vi "Get Project Paths.vi"(8 "error in (no error)":errorcluster, 11 "VI in":refnum<vi>) -> (0 "error out":errorcluster, 1 "project errors path":path, 2 "project path":path, 3 "VI out":refnum<vi>)   [LabVIEW 2017]
doc: "Returns <b>project path</b> for the <b>VI in</b> owning project and project errors file path if such file exist. Errors file name format is: project_name-errors.txt"
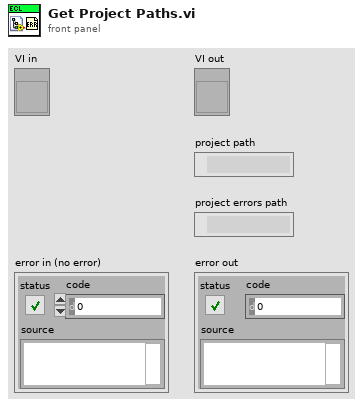
[diagram p1: front panel]
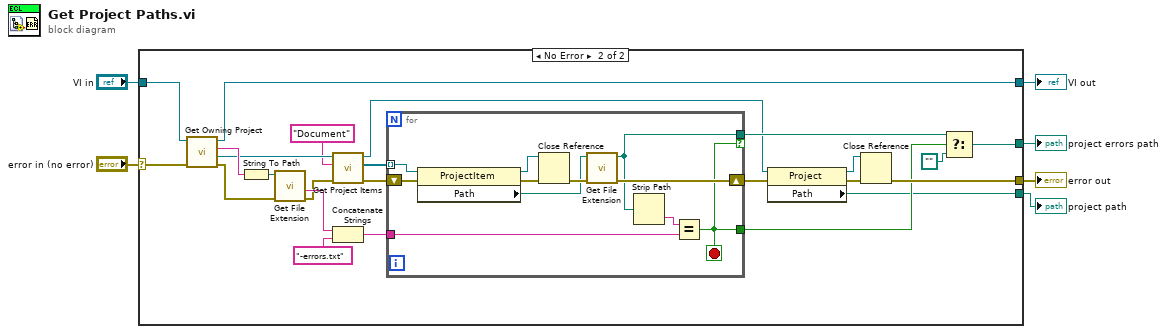
[diagram p0: block diagram]
diagram:
  n1 = case shown="No Error" "error in (no error)" {
    selector: "error in (no error)" -> [w8 w22]
    tunnel: [w8 w23] -> w5
    tunnel: [w7 w21] -> w4
    tunnel: "VI in" -> [w7 w20]
    tunnel: [_ w17] -> w2
    tunnel: [_ w10] -> w1
    frame Error {
    }
    frame No Error {
      n2 = call "Get Owning Project.vi"("error in (no error)"=w22, "VI in"=w20) -> ("error out"=w31:errorcluster, "owning project ref"=w15:refnum<vi>, "owning project name"=w28:string, "VI out"=w21:refnum<vi>)  [unwired: 6 in]
      n3 = String To Path(string=w28) -> (path=w29:path)
      n4 = call <vilib>:"Get File Extension.vi"("error in (no error)"=w31, "file"=w29) -> ("error out"=w24:errorcluster, "filename without extension"=w30:string)  [unwired: 5 in, 3 out]
      n5 = call "Get Project Items.vi"("error in (no error)"=w24, "type"="Document", "project in"=w15) -> ("error out"=w27:errorcluster, "project items"=w32:refnum<vi>[], "project out"=w13:refnum<vi>)  [unwired: 6 in]
      n6 = Concatenate Strings(w30, "-errors.txt" ("string")) -> (w26:string)
      n7 = for {
        tunnel: w26 -> [w40]
        shift-right: [w43] -> w14
        shift-left: w27 -> [w39]
        tunnel: [w34] -> w18 if=w36
        tunnel: [w36] -> w19
        tunnel: w32 -> [w35] mode=indexing
        stop <- w36 stop-if-true
        n8 = property class="ProjectItem"(reference=w35, error in=w39) -> (reference out=w37:refnum<vi>, error out=w38:errorcluster, "Path"=w41:path)
        n9 = Close Reference(reference=w37, error in (no error)=w38) -> (error out=w42:errorcluster)
        n10 = call <vilib>:"Get File Extension.vi"("error in (no error)"=w42, "file"=w41) -> ("error out"=w43:errorcluster, "dup file"=w34:path)  [unwired: 5 in, 3 out]
        n11 = Strip Path(path=w34) -> (name=w33:string)  [unwired: 1 out]
        n12 = Equal?(x=w33, y=w40) -> (x = y?=w36:bool)
      }
      n13 = property class="Project"(reference=w13, error in=w14) -> (reference out=w12:refnum<vi>, error out=w11:errorcluster, "Path"=w10:path)
      n14 = Close Reference(reference=w12, error in (no error)=w11) -> (error out=w23:errorcluster)
      n15 = Select(t=w18, s=w19, f=path "") -> (s? t:f=w17:path)
    }
  }
  "error out" <- w5
  "VI out" <- w4
  "project errors path" <- w2
  "project path" <- w1
